vi "Event.vi"(7 "Actor in":refnum<class "Actor.lvclass">, 11 "Event in":refnum<class "Event.lvclass">) -> (5 "Actor out":refnum<class "Actor.lvclass">)   [LabVIEW 2021, in "Event.lvclass"]
uses:
  Event.lvclass
  Actor/Actor.lvclass
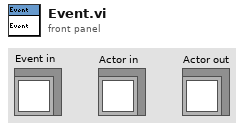
[diagram p1: front panel]
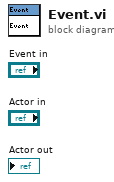
[diagram p0: block diagram]
diagram:
